vi "EOMSetPosition.vi"(0 "value":sgl format="%.2f") -> ()   [LabVIEW 2009]
uses:
  AO Update Channel (scaled value).vi
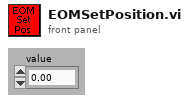
[diagram p1: front panel]
types:
  T1 = typedef "AnalogSettings.ctt" = cluster{"PCI 671x Device Number":u32, "Samples per Unit":u32}
  T2 = typedef "EOMSettings.ctt" = cluster{"Output Channel":tag, "EOM Voltage":dbl, "Pixel per Polymode Cycle":u32, "Time per Polymode Cycle":dbl}
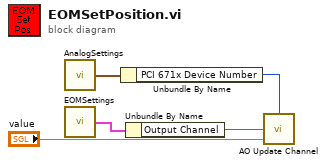
[diagram p0: block diagram]
diagram:
  n1 = call "AnalogSettings.vi"() -> ("Analog Settings (output)"=w2:T1)  [unwired: 2 in]
  n2 = call "EOMSettings.vi"() -> ("EOM Settings (output)"=w3:T2)  [unwired: 2 in]
  n3 = Unbundle By Name(w2) -> ("PCI 671x Device Number"=w1:u32)
  n4 = Unbundle By Name(w3) -> ("Output Channel"=w4:tag)
  n5 = call-poly "AO Update Channel.vi"("value"="value", "channel (0)"=w4, "device"=w1) -> ()
